vi "gen_node.vi"(10 "Name and Type":T3(array[cluster])) -> (2 "Block Data Array":T4[](array[typedef]) {"Terminal Flags" format="%.0b"})   [LabVIEW 2018]
uses:
  <vilib>/BlockNodeSupport/TerminalData.ctl
  StudioHelper/Gtor/Mth/GenVI/Intf/GenStdVI/Mth/GenOneStdVI/TypeDefinitions/control_data_type.ctl
panel:
  in  "z_Enum":enum16{""}(ring)
  in  "y_Enum":enum16{""}(ring)
  in  "x_Enum":enum16{""}(ring)
  in  "w_Enum":enum16{""}(ring)
  in  "v_Enum":enum16{""}(ring)
  in  "u_Enum":enum16{""}(ring)
  in  "t_Enum":enum16{""}(ring)
  in  "s_Enum":enum16{""}(ring)
  in  "r_Enum":enum16{""}(ring)
  in  "q_Enum":enum16{""}(ring)
  in  "p_Enum":enum16{""}(ring)
  in  "o_Enum":enum16{""}(ring)
  in  "n_Enum":enum16{""}(ring)
  in  "m_Enum":enum16{""}(ring)
  in  "l_Enum":enum16{""}(ring)
  in  "k_Enum":enum16{""}(ring)
  in  "j_Enum":T1(ring)
  in  "i_Enum":enum16{"MODE", "USER", "LAST", "PRES"}(ring)
  in  "h_Enum":enum16{""}(ring)
  in  "g_Enum":enum16{""}(ring)
  in  "f_Enum":enum16{"ALL", "NRF"}(ring)
  in  "d_Enum":enum16{"ON", "PART", "OFF"}(ring)
  in  "e_Enum":enum16{"ON", "PART", "OFF"}(ring)
  in  "c_Enum":enum16{""}(ring)
  in  "a_Enum":enum16{"1.2", "1.3"}(ring)
  in  "b_Enum":enum16{"OFF", "ON"}(ring)
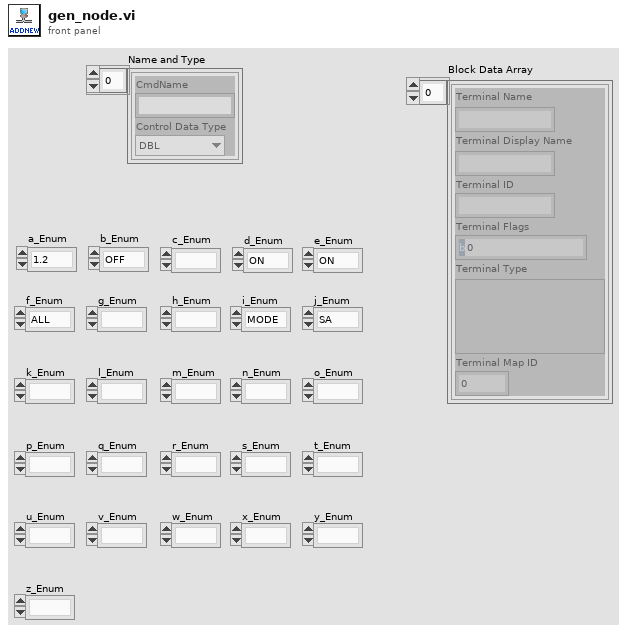
[diagram p1: front panel]
types:
  T1 = enum16{"SA", "BASIC", "ADEMOD", "NFIGURE", "PNOISE", "CDMA2K", "TDSCDMA", "VSA", "VSA89601", "WCDMA", "WIMAXOFDMA"}
  T2 = typedef "control_data_type.ctl" = enum16{"DBL", "I32", "Boolean", "String", "U16", "U32", "EXT", "SGL", "I16", "U8", "I8", "I64", "U64", "Waveform", "Reference", "Variant", "Cluster"}
  T3 = cluster{"CmdName":string, "Control Data Type":T2}[]
  T4 = typedef "TerminalData.ctl" = cluster{"Terminal Name":string, "Terminal Display Name":string, "Terminal ID":string, "Terminal Flags":i32, "Terminal Type":variant, "Terminal Map ID":i32}
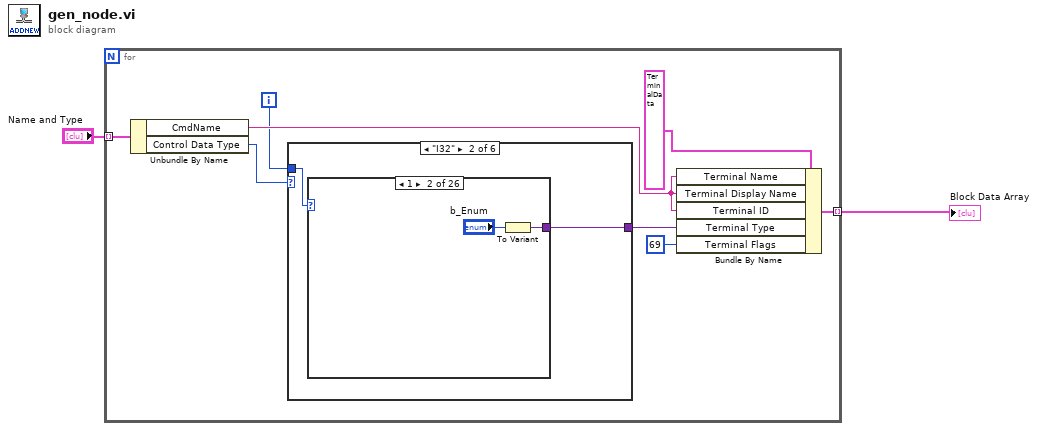
[diagram p0: block diagram]
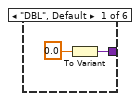
[diagram p2: hidden frame]
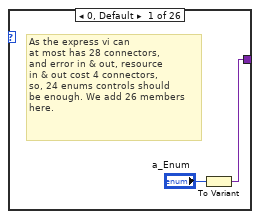
[diagram p3: hidden frame]
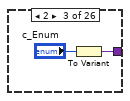
[diagram p4: hidden frame]
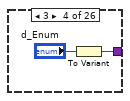
[diagram p5: hidden frame]
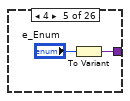
[diagram p6: hidden frame]
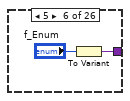
[diagram p7: hidden frame]
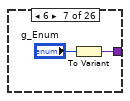
[diagram p8: hidden frame]
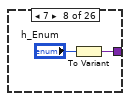
[diagram p9: hidden frame]
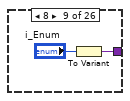
[diagram p10: hidden frame]
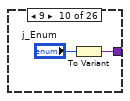
[diagram p11: hidden frame]
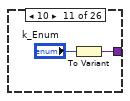
[diagram p12: hidden frame]
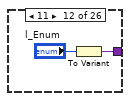
[diagram p13: hidden frame]
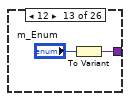
[diagram p14: hidden frame]
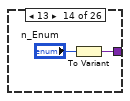
[diagram p15: hidden frame]
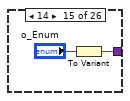
[diagram p16: hidden frame]
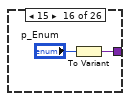
[diagram p17: hidden frame]
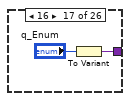
[diagram p18: hidden frame]
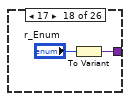
[diagram p19: hidden frame]
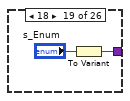
[diagram p20: hidden frame]
diagram:
  n1 = for {
    tunnel: [w9] -> w1 mode=indexing
    tunnel: "Name and Type" -> [w6] mode=indexing
    i -> [w3]
    n2 = Unbundle By Name(w6) -> ("CmdName"=w4:string, "Control Data Type"=w5:T2)
    n3 = case shown="\"I32\"" w5 {
      tunnel: [w11 w13 w67 w69 w71 w73] -> w7
      tunnel: w3 -> [_ w14 _ _ _ _]
      frame "DBL", Default {
        n4 = To Variant(anything=0.0) -> (Variant=w11:variant)
      }
      frame "I32" {
        n5 = case shown="1" w14 {
          tunnel: [w16 w18 w20 w22 w24 w25 w27 w30 w31 w33 w35 w37 w39 w41 w43 w45 w47 w49 w51 w54 w55 w57 w59 w61 w63 w65] -> w13
          frame 0, Default {
            # "As the express vi can\nat most has 28 connectors,\nand error in & out, resource \nin & out cost 4 connectors,\nso, 24 enums controls should\nbe enough. We add 26 members\nhere."
            n6 = To Variant(anything="a_Enum") -> (Variant=w16:variant)
          }
          frame 1 {
            n7 = To Variant(anything="b_Enum") -> (Variant=w18:variant)
          }
          frame 2 {
            n8 = To Variant(anything="c_Enum") -> (Variant=w20:variant)
          }
          frame 3 {
            n9 = To Variant(anything="d_Enum") -> (Variant=w22:variant)
          }
          frame 4 {
            n10 = To Variant(anything="e_Enum") -> (Variant=w24:variant)
          }
          frame 5 {
            n11 = To Variant(anything="f_Enum") -> (Variant=w25:variant)
          }
          frame 6 {
            n12 = To Variant(anything="g_Enum") -> (Variant=w27:variant)
          }
          frame 7 {
            n13 = To Variant(anything="h_Enum") -> (Variant=w30:variant)
          }
          frame 8 {
            n14 = To Variant(anything="i_Enum") -> (Variant=w31:variant)
          }
          frame 9 {
            n15 = To Variant(anything="j_Enum") -> (Variant=w33:variant)
          }
          frame 10 {
            n16 = To Variant(anything="k_Enum") -> (Variant=w35:variant)
          }
          frame 11 {
            n17 = To Variant(anything="l_Enum") -> (Variant=w37:variant)
          }
          frame 12 {
            n18 = To Variant(anything="m_Enum") -> (Variant=w39:variant)
          }
          frame 13 {
            n19 = To Variant(anything="n_Enum") -> (Variant=w41:variant)
          }
          frame 14 {
            n20 = To Variant(anything="o_Enum") -> (Variant=w43:variant)
          }
          frame 15 {
            n21 = To Variant(anything="p_Enum") -> (Variant=w45:variant)
          }
          frame 16 {
            n22 = To Variant(anything="q_Enum") -> (Variant=w47:variant)
          }
          frame 17 {
            n23 = To Variant(anything="r_Enum") -> (Variant=w49:variant)
          }
          frame 18 {
            n24 = To Variant(anything="s_Enum") -> (Variant=w51:variant)
          }
          frame 19 {
            n25 = To Variant(anything="t_Enum") -> (Variant=w54:variant)
          }
          frame 20 {
            n26 = To Variant(anything="u_Enum") -> (Variant=w55:variant)
          }
          frame 21 {
            n27 = To Variant(anything="v_Enum") -> (Variant=w57:variant)
          }
          frame 22 {
            n28 = To Variant(anything="w_Enum") -> (Variant=w59:variant)
          }
          frame 23 {
            n29 = To Variant(anything="x_Enum") -> (Variant=w61:variant)
          }
          frame 24 {
            n30 = To Variant(anything="y_Enum") -> (Variant=w63:variant)
          }
          frame 25 {
            n31 = To Variant(anything="z_Enum") -> (Variant=w65:variant)
          }
        }
      }
      frame "Boolean" {
        n32 = To Variant(anything=FALSE ("x")) -> (Variant=w67:variant)
      }
      frame "String" {
        n33 = To Variant(anything="") -> (Variant=w69:variant)
      }
      frame "U16" {
        n34 = To Variant(anything=0 ("Terminal Flags")) -> (Variant=w71:variant)
      }
      frame "U32" {
        n35 = To Variant(anything=0 ("Terminal Flags")) -> (Variant=w73:variant)
      }
    }
    n36 = Bundle By Name(cluster=T4 {"Terminal Name"="", "Terminal Display Name"="", "Terminal ID"="", "Terminal Flags"=0, "Terminal Type"=variant, "Terminal Map ID"=0} ("deleted portion"), "Terminal Name"=w4, "Terminal Display Name"=w4, "Terminal ID"=w4, "Terminal Type"=w7, "Terminal Flags"=69) -> (w9:T4)
  }
  "Block Data Array" <- w1
